vi "Telescope Init.vi"(8 "error in (no error)":errorcluster, 9 "Settings":variant, 10 "Name":string, 11 "Telescope in":refnum<class "Telescope.lvclass">) -> (0 "error out":errorcluster, 1 "Connect Message":string, 2 "Channel List":refnum<class "HK Item.lvclass">[](array[class]), 3 "Telescope out":refnum<class "Telescope.lvclass">)   [LabVIEW 2024, in "Telescope.lvclass"]
uses:
  Telescope.lvclass
  hk-channel-class/hk-channel-class/HK Item/HK Item.lvclass
  Telescope cluster Status.ctl
  typedefs/CC cluster RA and DEC.ctl
  Telescope enum Status.ctl
  Telescope.lvclass/Telescope.ctl
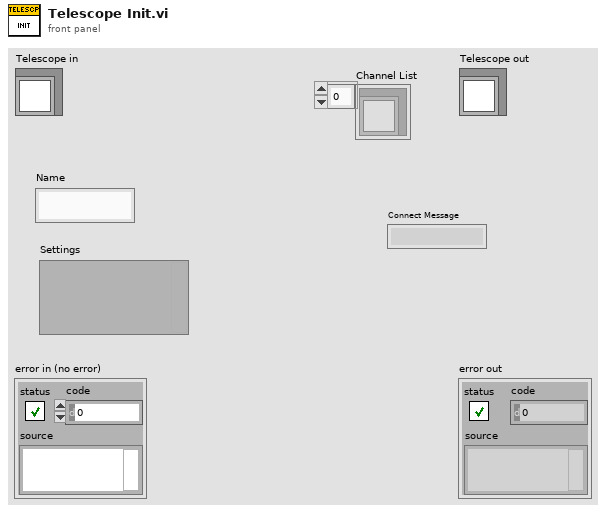
[diagram p1: front panel]
types:
  T1 = typedef "Telescope.lvclass/Telescope cluster Status.ctl" = cluster{"Position":T2, "Connected":bool, "Status":T3, "Curr Time":timestamp, "Status Word":u32, "Focus Pos A":dbl, "UTC Time":timestamp, "Local Sidreal Time":dbl, "Azimuth":dbl, "Altitude":dbl, "Rotator Angle":dbl, "RA String":string, "DEC String":string, "secZ":dbl, "Focus Pos B":dbl, "Focus Pos A-B":dbl, "Rotator Offset":dbl, "Time Offset":dbl, "Dome Angle":dbl, "Dome Status Word":u32, "Dome Moving":bool}
  T2 = typedef "CC cluster RA and DEC.ctl" = cluster{"RA":dbl, "DEC":dbl}
  T3 = typedef "Telescope.lvclass/Telescope enum Status.ctl" = enum16{"Initializing", "Ready", "Moving", "Focusing", "Error"}
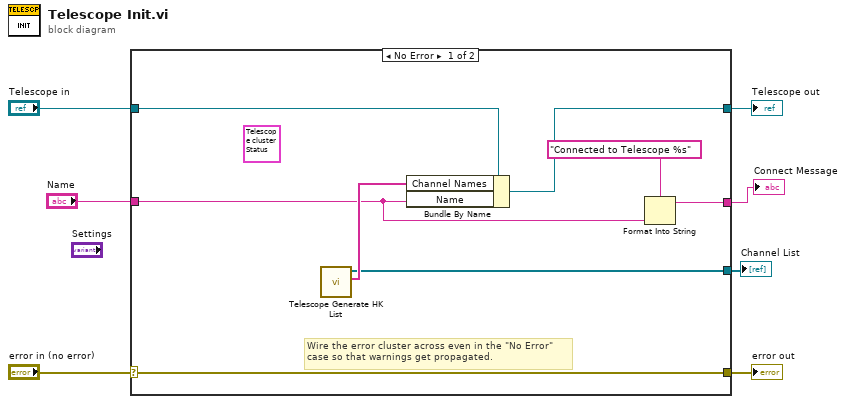
[diagram p0: block diagram]
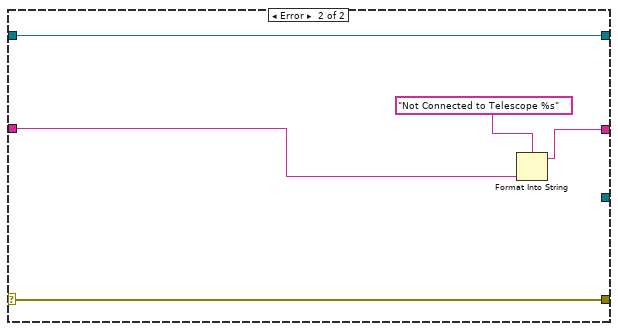
[diagram p2: hidden frame]
diagram:
  n1 = case shown="No Error" "error in (no error)" {
    selector: "error in (no error)" -> [w15 w20]
    tunnel: [w15 w20] -> w6
    tunnel: [w14 w19] -> w4
    tunnel: "Telescope in" -> [w13 w19]
    tunnel: "Name" -> [w10 w16]
    tunnel: [w9 w17] -> w2
    tunnel: [w8 _] -> w1
    frame No Error {
      (unwired) T1 {"Position"={"RA"=0.0, "DEC"=0.0}, "Connected"=FALSE, "Status"=enum."Initializing", "Curr Time"=timestamp(0 s since 1904-01-01), "Status Word"=0, "Focus Pos A"=0.0, "UTC Time"=timestamp(0 s since 1904-01-01), "Local Sidreal Time"=0.0, "Azimuth"=0.0, "Altitude"=0.0, "Rotator Angle"=0.0, "RA String"="", "DEC String"="", "secZ"=0.0, "Focus Pos B"=0.0, "Focus Pos A-B"=0.0, "Rotator Offset"=0.0, "Time Offset"=0.0, "Dome Angle"=0.0, "Dome Status Word"=0, "Dome Moving"=FALSE} ("Telescope Status")
      # "Wire the error cluster across even in the \"No Error\"\ncase so that warnings get propagated."
      n2 = call "Telescope Generate HK List.vi"() -> ("Channel Names"=w12:string[], "Channel List"=w8:refnum<class "HK Item.lvclass">[])  [unwired: 10 in]
      n3 = Bundle By Name(cluster=w13, "Channel Names"=w12, "Name"=w10) -> (w14:refnum<class "Telescope.lvclass">)
      n4 = Format Into String(format string="Connected to Telescope %s", w10) -> (resulting string=w9:string)  [unwired: 2 in, 1 out]
    }
    frame Error {
      n5 = Format Into String(format string="Not Connected to Telescope %s", w16) -> (resulting string=w17:string)  [unwired: 2 in, 1 out]
    }
  }
  "error out" <- w6
  "Telescope out" <- w4
  "Channel List" <- w1
  "Connect Message" <- w2
